vi "VI Tree.vi"   [LabVIEW 2015, in "Agilent 3352X Series.lvlib"]
doc: "This is the instrument driver for the Agilent 3352X. It includes 33500 series models and 33600 series models. The VI Tree displays all the user-callable VIs of the instrument driver in an organized table."
uses:
  <instrlib>/Agilent 3352X Series/Agilent 3352X Series.lvlib
  <instrlib>/Agilent 3352X Series/Public/Configure/Configure Standard Waveform Advanced (Pulse).vi
  <instrlib>/Agilent 3352X Series/Public/Configure/Modulation/Configure Modulation (Amplitude).vi
panel:
  # "(c) 2011 - 2015 National Instruments.  ALL RIGHTS RESERVED."
  # "SEE DIAGRAM\nFOR VI TREE."
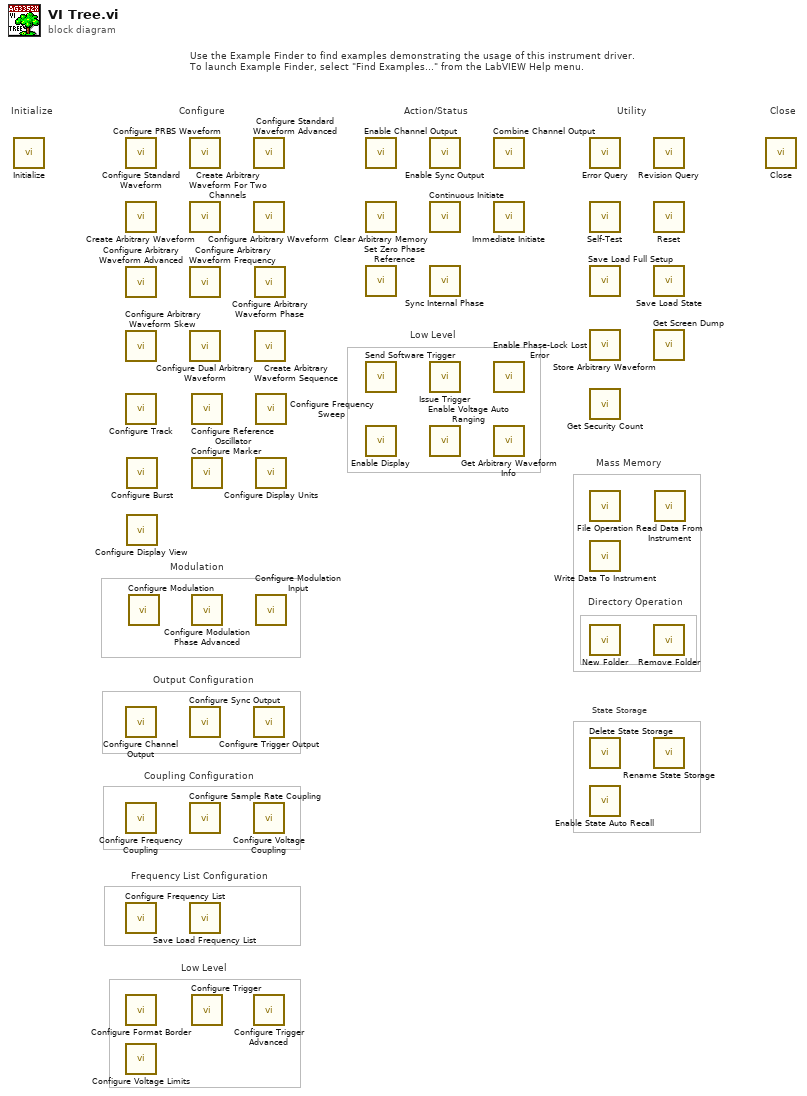
[diagram p0: block diagram]
diagram:
  # "Directory Operation"
  # "State Storage"
  # "Mass Memory"
  # "Frequency List Configuration"
  # "Coupling Configuration"
  # "Output Configuration"
  # "Modulation"
  # "Low Level"
  # "Low Level"
  # "Use the Example Finder to find examples demonstrating the usage of this instrument driver.\nTo launch Example Finder, select \"Find Examples...\" from the LabVIEW Help menu."
  # "Configure"
  # "Utility"
  # "Action/Status"
  # "Close"
  # "Initialize"
  n1 = call <instrlib>:"Initialize.vi"() -> ()  [unwired: 10 in, 2 out]
  n2 = call <instrlib>:"Configure Standard Waveform.vi"() -> ()  [unwired: 14 in, 2 out]
  n3 = call <instrlib>:"Create Arbitrary Waveform.vi"() -> ()  [unwired: 10 in, 2 out]
  n4 = call <instrlib>:"Configure Arbitrary Waveform Advanced.vi"() -> ()  [unwired: 10 in, 2 out]
  n5 = call <instrlib>:"Configure Arbitrary Waveform Skew.vi"() -> ()  [unwired: 10 in, 2 out]
  n6 = call <instrlib>:"Configure Track.vi"() -> ()  [unwired: 10 in, 2 out]
  n7 = call <instrlib>:"Configure Channel Output.vi"() -> ()  [unwired: 14 in, 2 out]
  n8 = call <instrlib>:"Configure Frequency Coupling.vi"() -> ()  [unwired: 10 in, 2 out]
  n9 = call <instrlib>:"Configure Frequency List.vi"() -> ()  [unwired: 10 in, 2 out]
  n10 = call <instrlib>:"Configure Format Border.vi"() -> ()  [unwired: 10 in, 2 out]
  n11 = call <instrlib>:"Configure Voltage Limits.vi"() -> ()  [unwired: 10 in, 2 out]
  n12 = call <instrlib>:"Configure Burst.vi"() -> ()  [unwired: 14 in, 2 out]
  n13 = call <instrlib>:"Configure Display View.vi"() -> ()  [unwired: 10 in, 2 out]
  n14 = call-poly <instrlib>:"Configure Modulation.vi"() -> ()  [unwired: 14 in, 2 out]
  n15 = call <instrlib>:"Configure PRBS Waveform.vi"() -> ()  [unwired: 10 in, 2 out]
  n16 = call <instrlib>:"Create Arbitrary Waveform For Two Channels.vi"() -> ()  [unwired: 10 in, 2 out]
  n17 = call <instrlib>:"Configure Arbitrary Waveform Frequency.vi"() -> ()  [unwired: 10 in, 2 out]
  n18 = call <instrlib>:"Configure Dual Arbitrary Waveform.vi"() -> ()  [unwired: 10 in, 2 out]
  n19 = call <instrlib>:"Configure Sync Output.vi"() -> ()  [unwired: 10 in, 2 out]
  n20 = call <instrlib>:"Configure Sample Rate Coupling.vi"() -> ()  [unwired: 14 in, 2 out]
  n21 = call <instrlib>:"Save Load Frequency List.vi"() -> ()  [unwired: 10 in, 2 out]
  n22 = call <instrlib>:"Configure Reference Oscillator.vi"() -> ()  [unwired: 10 in, 2 out]
  n23 = call <instrlib>:"Configure Marker.vi"() -> ()  [unwired: 10 in, 2 out]
  n24 = call <instrlib>:"Configure Modulation Phase Advanced.vi"() -> ()  [unwired: 10 in, 2 out]
  n25 = call <instrlib>:"Configure Trigger.vi"() -> ()  [unwired: 10 in, 2 out]
  n26 = call-poly <instrlib>:"Configure Standard Waveform Advanced.vi"() -> ()  [unwired: 10 in, 2 out]
  n27 = call <instrlib>:"Configure Arbitrary Waveform.vi"() -> ()  [unwired: 14 in, 2 out]
  n28 = call <instrlib>:"Configure Trigger Output.vi"() -> ()  [unwired: 10 in, 2 out]
  n29 = call <instrlib>:"Configure Voltage Coupling.vi"() -> ()  [unwired: 10 in, 2 out]
  n30 = call <instrlib>:"Configure Trigger Advanced.vi"() -> ()  [unwired: 10 in, 2 out]
  n31 = call <instrlib>:"Configure Arbitrary Waveform Phase.vi"() -> ()  [unwired: 10 in, 2 out]
  n32 = call <instrlib>:"Create Arbitrary Waveform Sequence.vi"() -> ()  [unwired: 10 in, 2 out]
  n33 = call <instrlib>:"Configure Frequency Sweep.vi"() -> ()  [unwired: 14 in, 2 out]
  n34 = call <instrlib>:"Configure Display Units.vi"() -> ()  [unwired: 10 in, 2 out]
  n35 = call <instrlib>:"Configure Modulation Input.vi"() -> ()  [unwired: 10 in, 2 out]
  n36 = call <instrlib>:"Enable Channel Output.vi"() -> ()  [unwired: 10 in, 2 out]
  n37 = call <instrlib>:"Clear Arbitrary Memory.vi"() -> ()  [unwired: 10 in, 2 out]
  n38 = call <instrlib>:"Set Zero Phase Reference.vi"() -> ()  [unwired: 10 in, 2 out]
  n39 = call <instrlib>:"Send Software Trigger.vi"() -> ()  [unwired: 10 in, 2 out]
  n40 = call <instrlib>:"Enable Display.vi"() -> ()  [unwired: 10 in, 2 out]
  n41 = call <instrlib>:"Enable Sync Output.vi"() -> ()  [unwired: 10 in, 2 out]
  n42 = call <instrlib>:"Continuous Initiate.vi"() -> ()  [unwired: 10 in, 2 out]
  n43 = call <instrlib>:"Sync Internal Phase.vi"() -> ()  [unwired: 10 in, 2 out]
  n44 = call <instrlib>:"Issue Trigger.vi"() -> ()  [unwired: 10 in, 2 out]
  n45 = call <instrlib>:"Enable Voltage Auto Ranging.vi"() -> ()  [unwired: 10 in, 2 out]
  n46 = call <instrlib>:"Combine Channel Output.vi"() -> ()  [unwired: 10 in, 2 out]
  n47 = call <instrlib>:"Immediate Initiate.vi"() -> ()  [unwired: 10 in, 2 out]
  n48 = call <instrlib>:"Enable Phase-Lock Lost Error.vi"() -> ()  [unwired: 10 in, 2 out]
  n49 = call <instrlib>:"Get Arbitrary Waveform Info.vi"() -> ()  [unwired: 9 in, 3 out]
  n50 = call <instrlib>:"Error Query.vi"() -> ()  [unwired: 8 in, 4 out]
  n51 = call <instrlib>:"Self-Test.vi"() -> ()  [unwired: 8 in, 4 out]
  n52 = call <instrlib>:"Save Load Full Setup.vi"() -> ()  [unwired: 10 in, 2 out]
  n53 = call <instrlib>:"Store Arbitrary Waveform.vi"() -> ()  [unwired: 10 in, 2 out]
  n54 = call <instrlib>:"Get Security Count.vi"() -> ()  [unwired: 9 in, 3 out]
  n55 = call <instrlib>:"File Operation.vi"() -> ()  [unwired: 10 in, 2 out]
  n56 = call <instrlib>:"Write Data To Instrument.vi"() -> ()  [unwired: 10 in, 2 out]
  n57 = call <instrlib>:"New Folder.vi"() -> ()  [unwired: 10 in, 2 out]
  n58 = call <instrlib>:"Delete State Storage.vi"() -> ()  [unwired: 10 in, 2 out]
  n59 = call <instrlib>:"Enable State Auto Recall.vi"() -> ()  [unwired: 10 in, 2 out]
  n60 = call <instrlib>:"Revision Query.vi"() -> ()  [unwired: 8 in, 4 out]
  n61 = call <instrlib>:"Reset.vi"() -> ()  [unwired: 10 in, 2 out]
  n62 = call <instrlib>:"Save Load State.vi"() -> ()  [unwired: 10 in, 2 out]
  n63 = call <instrlib>:"Get Screen Dump.vi"() -> ()  [unwired: 10 in, 2 out]
  n64 = call <instrlib>:"Remove Folder.vi"() -> ()  [unwired: 10 in, 2 out]
  n65 = call <instrlib>:"Rename State Storage.vi"() -> ()  [unwired: 10 in, 2 out]
  n66 = call <instrlib>:"Read Data From Instrument.vi"() -> ()  [unwired: 9 in, 3 out]
  n67 = call <instrlib>:"Close.vi"() -> ()  [unwired: 11 in, 1 out]
